vi "DisposeCore.vi"(8 "error in (no error)":errorcluster, 11 "CreatorA":refnum<class "CreatorA.lvclass">) -> (0 "error out":errorcluster, 3 "CreatorA":refnum<class "CreatorA.lvclass">)   [LabVIEW 2020, in "FactoryMethod.lvlib" / "FactoryMethodLazyEvaluation.lvlib" / "CreatorA.lvclass"]
uses:
  CreatorA.lvclass
  Private/TypeDef/privateDataDVR.ctl
  Private/TypeDef/privateData.ctl
  CreatorA.lvclass/CreatorA.ctl
  Creator/Creator.lvclass
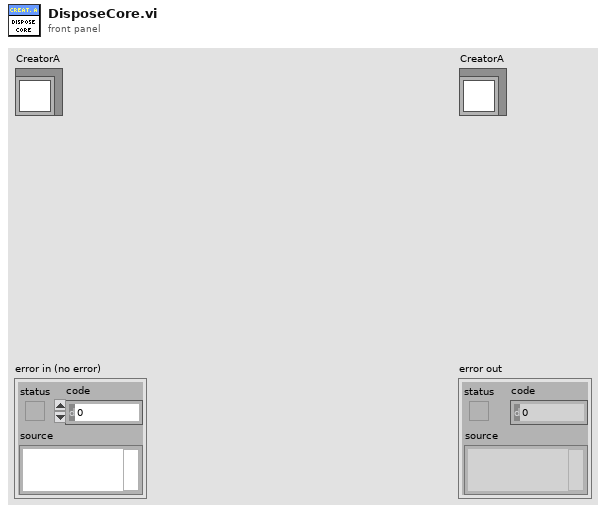
[diagram p1: front panel]
types:
  T1 = typedef "FactoryMethod.lvlib/FactoryMethodLazyEvaluation.lvlib/CreatorA.lvclass/privateDataDVR.ctl" = refnum<data-value>
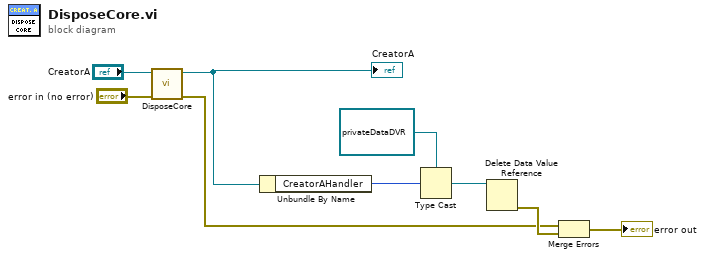
[diagram p0: block diagram]
diagram:
  n1 = call-parent "DisposeCore.vi"("error in (no error)"="error in (no error)", "Creator in"="CreatorA") -> ("error out"=w2:errorcluster, "Creator out"=w1:refnum<class "CreatorA.lvclass">)  [unwired: 8 in]
  "CreatorA" <- w1
  n2 = Unbundle By Name(w1) -> ("CreatorAHandler"=w6:u32)
  n3 = Type Cast(type=T1 refnum ("privateDataDVR"), x=w6) -> (*(type *) &x=w7:T1)
  n4 = Delete Data Value Reference(data value reference=w7) -> (error out=w4:errorcluster)  [unwired: 1 in, 1 out]
  n5 = Merge Errors(w2, w4) -> (→"error out":errorcluster)
